vi "Write Event Data.vi"(10 "Event Actors.lvlib:Event":refnum<class "Event.lvclass">, 11 "Abstract Event Message for View in":refnum<class "Abstract Event Message for View.lvclass">) -> (3 "Abstract Event Message for View out":refnum<class "Abstract Event Message for View.lvclass">)   [LabVIEW 2017, in "Event Actors.lvlib" / "Abstract Event Message for View.lvclass"]
uses:
  Abstract Event Message for View.lvclass
  Event/Event.lvclass
  Abstract Event Message for View.lvclass/Abstract Event Message for View.ctl
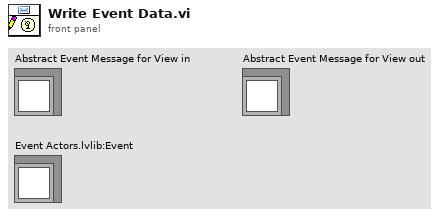
[diagram p1: front panel]
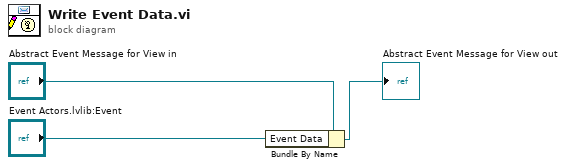
[diagram p0: block diagram]
diagram:
  n1 = Bundle By Name(cluster="Abstract Event Message for View in", "Event Data"="Event Actors.lvlib:Event") -> (→"Abstract Event Message for View out":refnum<class "Abstract Event Message for View.lvclass">)
